vi "20170502127惠雨1.vi"() -> ()   [LabVIEW 2017]
panel:
  out "布尔 7":bool
  out "布尔 6":bool
  out "布尔":bool
  out "布尔 2":bool
  out "布尔 3":bool
  out "布尔 4":bool
  out "布尔 5":bool
  in  "延时（s）":dbl(knob) scale=0.1..0.5
  in  "停止":bool
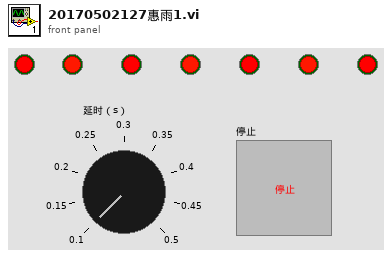
[diagram p1: front panel]
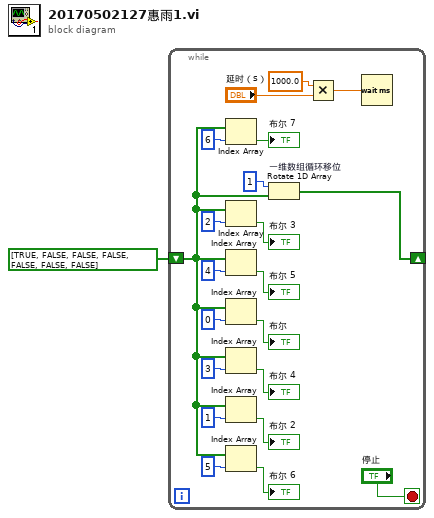
[diagram p0: block diagram]
diagram:
  n1 = while {
    shift-right: [w21] -> _
    shift-left: bool[] [TRUE, FALSE, FALSE, FALSE, FALSE, FALSE, FALSE] -> [w6]
    stop <- "停止" stop-if-true
    n2 = Index Array(array=w6, index=6 ("索引")) -> (element=→"布尔 7":bool)
    n3 = Index Array(array=w6, index=2 ("索引")) -> (element=→"布尔 3":bool)
    n4 = Index Array(array=w6, index=4 ("索引")) -> (element=→"布尔 5":bool)
    n5 = Index Array(array=w6, index=0 ("索引")) -> (element=→"布尔":bool)
    n6 = Index Array(array=w6, index=3 ("索引")) -> (element=→"布尔 4":bool)
    n7 = Index Array(array=w6, index=1 ("索引")) -> (element=→"布尔 2":bool)
    n8 = Index Array(array=w6, index=5 ("索引")) -> (element=→"布尔 6":bool)
    n9 = Rotate 1D Array "一维数组循环移位"(1:w6, 2:1 ("n")) -> (0:w21:bool[])
    n10 = Multiply(x=1000.0, y="延时（s）") -> (x*y=w7:dbl)
    n11 = Wait (ms)(milliseconds to wait=w7) -> ()  [unwired: 1 out]
  }
